vi "Get Stop Event.vi"(8 "error in (no error)":errorcluster, 11 "User Interface in":refnum<class "User Interface.lvclass">) -> (0 "error out":errorcluster, 2 "stop event":refnum<user-event>, 3 "User Interface out":refnum<class "User Interface.lvclass">)   [LabVIEW 2021, in "DSF Core.lvlib" / "User Interface.lvclass"]
uses:
  User Interface.lvclass
  User Interface Events/User Interface Events.lvclass
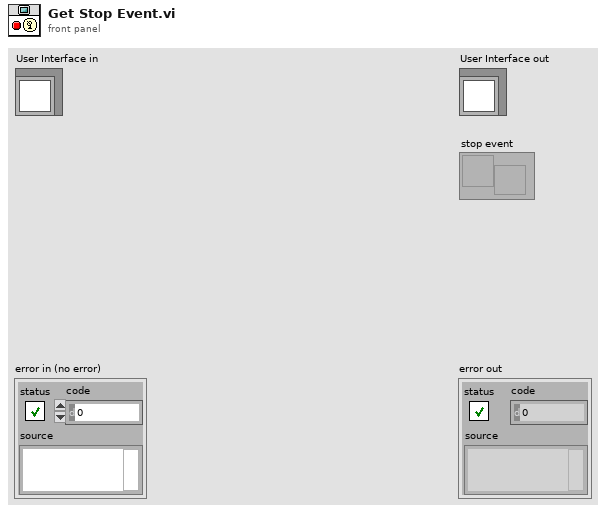
[diagram p1: front panel]
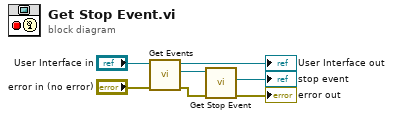
[diagram p0: block diagram]
diagram:
  n1 = call "Get Events.vi"("error in (no error)"="error in (no error)", "User Interface in"="User Interface in") -> ("error out"=w4:errorcluster, "events"=w3:refnum<class "User Interface Events.lvclass">, "User Interface out"=→"User Interface out":refnum<class "User Interface.lvclass">)  [unwired: 7 in]
  n2 = call "Get Stop Event.vi"("error in (no error)"=w4, "User Interface Events in"=w3) -> ("error out"=→"error out":errorcluster, "stop event"=→"stop event":refnum<user-event>)  [unwired: 7 in, 1 out]
